vi "write TBM configuration.vi"(8 "error in":errorcluster, 10 "configuration":refnum<class "TBM configuration.lvclass">, 11 "Asynchronous Module Editor Node in":refnum<class "Asynchronous Module Editor Node.lvclass">) -> (0 "error out":errorcluster, 3 "Asynchronous Module Editor Node out":refnum<class "Asynchronous Module Editor Node.lvclass">)   [LabVIEW 2013, in "PL Framework Configuration Tool.lvlib" / "Asynchronous Module Editor Node.lvclass"]
uses:
  Asynchronous Module Editor Node.lvclass
  <vilib>/NI/Tag Bus Module Framework/root configuration/TBM configuration.lvclass
  asynchronous execution module/configuration/asynchronous execution module configuration.lvclass
  Asynchronous Module Editor Node.lvclass/Asynchronous Module Editor Node.ctl
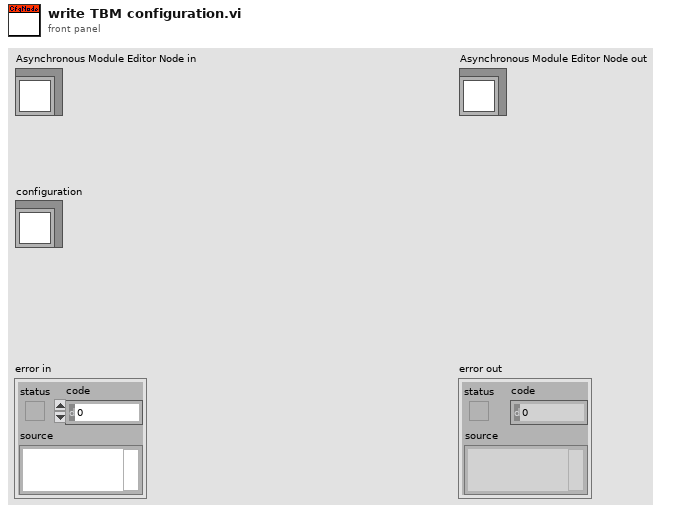
[diagram p1: front panel]
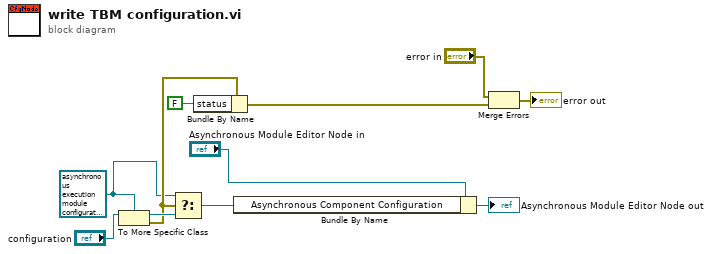
[diagram p0: block diagram]
diagram:
  w6 = refnum<class "asynchronous execution module configuration.lvclass"> refnum ("Asynchronous Component Configuration")
  n1 = To More Specific Class(target class=w6, reference="configuration") -> (specific class reference=w11:refnum<class "asynchronous execution module configuration.lvclass">, error out=w10:errorcluster)  [unwired: 1 in]
  n2 = Select(t=w6, s=w10, f=w11) -> (s? t:f=w7:refnum<class "asynchronous execution module configuration.lvclass">)
  n3 = Bundle By Name(cluster=w10, "status"=FALSE) -> (w8:errorcluster)
  n4 = Bundle By Name(cluster="Asynchronous Module Editor Node in", "Asynchronous Component Configuration"=w7) -> (→"Asynchronous Module Editor Node out":refnum<class "Asynchronous Module Editor Node.lvclass">)
  n5 = Merge Errors("error in", w8) -> (→"error out":errorcluster)
